vi "Calculate X Increment and Relative Initial X for Decimation.vi"(6 "Start Point (0)":i32, 7 "Actual Points (1000)":i32=1000, 9 "Original X Increment (0)":dbl, 10 "Original Relative Initial X (0)":dbl, 11 "Waveform Size (100)":i32=100) -> (1 "X Increment Out":dbl, 2 "Relative Initial X Out":dbl)   [LabVIEW 2020, in "Agilent 90000 Series.lvlib"]
doc: "Calculates the relative initial x and x increment for decimation."
uses:
  Agilent 90000 Series.lvlib
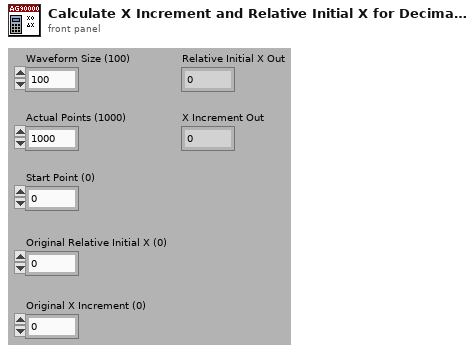
[diagram p1: front panel]
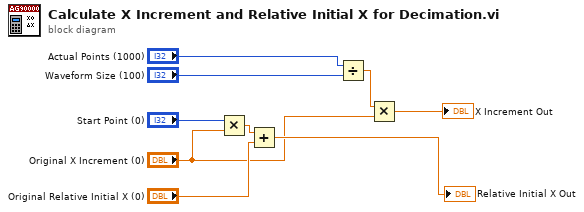
[diagram p0: block diagram]
diagram:
  n1 = Multiply(x="Start Point (0)", y="Original X Increment (0)") -> (x*y=w7:dbl)
  n2 = Add(x=w7, y="Original Relative Initial X (0)") -> (x+y=→"Relative Initial X Out":dbl)
  n3 = Divide(x="Actual Points (1000)", y="Waveform Size (100)") -> (x/y=w3:dbl)
  n4 = Multiply(x=w3, y="Original X Increment (0)") -> (x*y=→"X Increment Out":dbl)
